vi "main.vi"() -> ()   [LabVIEW 2019]
uses:
  <vilib>/addons/Control Design/_Model Construction/Data Typedefs.llb/CD frequency specs.ctl
  <vilib>/addons/Control Design/_Frequency Response Analysis/Frequency Response.llb/Frequency Response subVI/cd_Bode (State Space).vi
  <vilib>/addons/Control Design/_Frequency Response Analysis/NI_CD_Frequency Response.lvlib
  <vilib>/addons/Control Design/_Model Construction/NI_LinSys_Data Typedefs.lvlib
panel:
  in  "As":dbl=5.0 caption="Амплитуда сигнала, As"
  out "АЧХ, вычисленный вручную":cluster{"Frequency":dbl[], dbl[]}(graph)
  out "Искомый массив частот":dbl[](array[numeric])=[1.0, 1.0473708979594496, 1.0969857978923836, 1.1489510001873091, 1.20337784077759, 1.2603829296797278, 1.3200884008314184, 1.3826221737646567, 1.4481182276745346, 1.5167168884709241, 1.5885651294280543, 1.6638168860761304, 1.7426333860096521, 1.8251834943190455, 1.9116440753857047, 2.0022003718155874, 2.0970464013232357, 2.1963853724165494, 2.3004301197729218, 2.409403560239529, 2.5235391704347703, 2.6430814869741095, 2.7682866303920703, 2.8994228538828817, 3.036771118035464, 3.180625692794125, 3.331294787934679, 3.489101213406779, 3.654383070957264, 3.8274944785163205, 4.008806328898474, 4.198707084443918, 4.397603609302729, 4.605922041145116, 4.824108704165382, 5.052631065335692, 5.291978735958455, 5.54266452066312, 5.805225516094915, 6.08022426164944, 6.368249944718606, 6.669919663030142, 6.98587974678527, 7.31680714342722, 7.663410868007483, 8.026433522257202, 8.406652885618355, 8.804883581643494, 9.22197882333436, 9.65883224115874, 10.11637979766211, 10.5956017927762, 11.097524964120764, 11.623224686798574, 12.173827277396665, 12.750512407130188, 13.354515629299048, 13.987131026472447, 14.649713983072926, 15.343684089300197, 16.070528182616467, 16.83180353330965, 17.629141180959564, 18.46424942895553, 19.33891750455241, 20.255019392306775, 21.21451784910641, 22.219468609395356, 23.272024789604217, 24.37444150122234, 25.529080682395318, 26.738416158399623, 28.005038941836467, 29.331662783900615, 30.721129988617754, 30.997000000000003, 32.176417502507555, 33.700643292719484, 35.29707302730671, 36.969127071950496, 38.72038781812579, 40.16172070631751, 40.32654463353467, 40.49204499907432, 40.55460735840854, 40.65822457904315, 40.82508616094098, 40.99263254370755, 41.160866537769486, 41.32979096508739, 41.499408659203226, 41.669722465287826, 41.840735240188614, 42.01244985247753, 42.18486918249916, 42.357996122419046, 42.47571552536925, 42.53183357627216, 42.706384460011684, 42.88165170155787, 43.05763824084719, 43.23434702988161, 43.41178103277815, 43.58994322581855, 43.76883659749926, 43.94846414858153, 44.12882889214174, 44.30993385362195, 44.48782831127613, 44.491782070880674, 44.67437659424378, 44.85772048655573, 45.04181682323088, 45.226668692305125, 45.41227919448768, 45.598651443213065, 45.78578856469338, 45.973693697970695, 46.162369994969744, 46.351820620550775, 46.54204875256262, 46.595256686647105, 46.73305758189605, 46.92485031253724, 47.11743016162157, 47.310800359487544, 47.504964149730995, 47.6999247892595, 47.895685548347, 48.09224971068864, 48.289620573455906, 48.48780144735186, 48.68679565666673, 48.80251583654462, 48.88660653933364, 49.087237446984595, 49.28869174500675, 49.4909728125988, 49.69408404282771, 49.8980288426856, 50.102810633146895, 50.30843284922574, 50.51489894003359, 50.72221236883706, 50.930376613116046, 51.114334834402, 51.13939516462204, 51.349271529436685, 51.56000922803062, 51.771611795322514, 51.984082780738355, 52.197425748271, 52.41164427653995, 52.62674195885138, 52.84272240325842, 53.05958923262166, 53.277346084669944, 53.495996612061354, 53.5356667741076, 53.71554448244452, 53.93599337852012, 54.15734699810265, 54.379609054182474, 54.60278327498806, 54.82687340404857, 55.051883200256626, 55.27781643793134, 55.50467690688171, 55.732468412470084, 55.96119477567605, 56.07169938205495, 56.1908598331605, 56.421467437330044, 56.65302145640156, 56.88552577446712, 57.11898429155914, 57.35340092371575, 57.58877960304659, 57.825124277798636, 58.062438912422536, 58.300727487639044, 58.539994000505814, 58.727866131895205, 58.780242464484466, 59.021476909507854, 59.263701382047735, 59.50691994518259, 59.751136678665794, 59.99635567899408, 60.24258105947626, 60.994, 61.509857885805424, 64.42363508721417, 67.4754405311074, 70.6718127392754, 74.01959996915694, 77.52597488629515, 81.19844993184068, 85.04489341802739, 89.07354638610502, 90.99100000000001, 93.2930402628475, 97.71241535346567, 102.34114021054606, 107.18913192051356, 112.2667773510822, 117.58495540521655, 120.988, 123.1550603292835, 128.98902612533183, 135.0993521198037, 141.4991297434587, 148.202070579887, 155.222535742706, 162.5755666443807, 170.27691722259138, 178.34308769319242, 186.7913599020798, 195.63983435170803, 204.90746898158642, 214.61411978584223, 224.78058335487444, 235.42864143224375, 246.58110758226243, 258.2618760682698, 270.4959730463159, 283.309610183935, 296.73024081888957, 310.7866187782041, 325.5088599835088, 340.9285069746843, 357.0785964900496, 373.99373024788326, 391.7101490809297, 410.2658105827232, 429.70047043208825, 450.0557675700542, 471.3753134116769, 493.7047852839051, 517.0920242896809, 541.5871378079527, 567.2426068492035, 594.1133984965093, 622.2570836730293, 651.7339604882491, 682.6071834272459, 714.9428986597652, 748.81038575901, 784.2822061337762, 821.4343584919513, 860.3464416684594, 901.1018251665116, 943.7878277775483, 988.4959046625692, 1035.3218432956735, 1084.3659686896222, 1135.7333583431182, 1189.5340673703329, 1245.8833642950221, 1304.9019780144174, 1366.716356462022, 1431.4589375234953, 1499.2684327860632, 1570.2901247293955, 1644.676177994683, 1722.5859653988068, 1804.1864093920938, 1889.6523396912323, 1979.166867853581, 2072.9217795953964, 2171.1179456945306, 2273.965752357956, 2381.685551976188, 2494.5081352303473, 2612.675225563361, 2736.439997074705, 2866.0676169482877, 3001.835813575628, 3144.0354715915405, 3292.9712550971935, 3448.962260405803, 3612.342699709479, 3783.462617131979, 3962.6886387015306, 4150.404757850531, 4347.013158125083, 4552.93507486701, 4768.611697714535, 4994.505115855208, 5231.099308056334, 5478.901179594018, 5738.441648302474, 6010.276782070467, 6294.988990221976, 6593.18827133364, 6905.513520162426, 7232.6338964836405, 7575.250258772024, 7934.096665797607, 8309.941949353515, 8703.591361485289, 9115.888299750955, 9547.716114208199, 9850.015, 9880.012, 9910.009, 9940.006, 9970.003, 10000.0]
  out "АЧХ":cluster{"W":dbl[], "Magnitude":dbl[]}[](graph)
  in  "t, [s]":dbl=1.0 caption="Время t, [s]"
  in  "An":dbl caption="Амплитуда шума, An"
  in  "dt [s]":dbl=0.001 caption="Шаг дискретизации dt [s]"
  in  "f, [Hz]":dbl=1.0 caption="Частота сигнала f, [Hz]"
  in  "f_cut":dbl=10.0 caption="Частота среза f_cut [Hz]"
  in  "dbs":dbl=120.0 caption="Пульсации в полосе\nпропускания dbs, [db]"
  in  "dbp":dbl=0.05 caption="Пульсации в полосе\nподавления dbp [db]"
  in  "n":i32=2 caption="Порядок фильтра n"
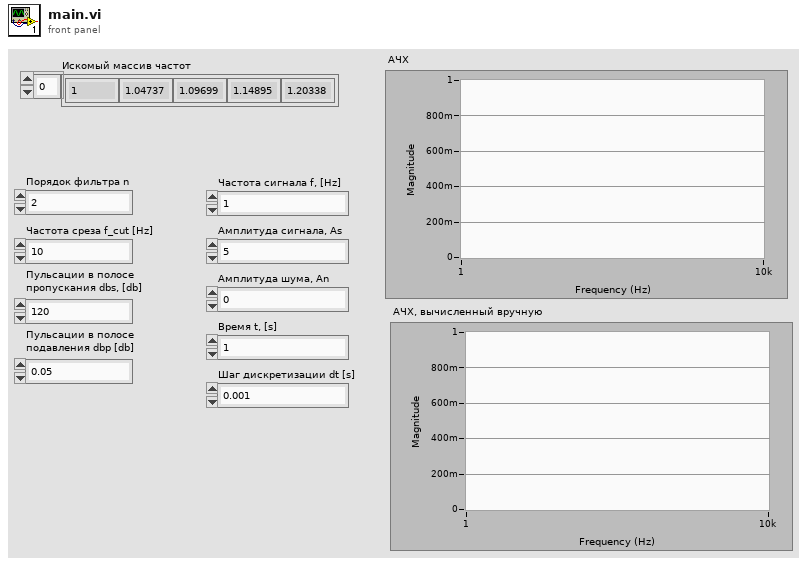
[diagram p1: front panel]
types:
  T1 = typedef "NI_LinSys_Data Typedefs.lvlib/CD frequency specs.ctl" = cluster{"Initial frequency":dbl, "Final frequency":dbl, "Minimum number of points":i32, "Frequency Unit":enum16{"Hz", "rad/s"}}
  T2 = typedef "NI_LinSys_Model Typedefs.lvlib/CD State Space Model (MIMO).ctl" = cluster{"properties":T3, "A":dbl[][], "B":dbl[][], "C":dbl[][], "D":dbl[][], "StateNames":string[], "Transport Delay":dbl[][]}
  T3 = typedef "NI_LinSys_Model Typedefs.lvlib/CD General Elements.ctl" = cluster{"Model name":string, "Input names":string[], "Output names":string[], "Input Delays":dbl[], "Output Delays":dbl[], "Sampling Time":dbl, "Notes":string}
  T4 = typedef "NI_LinSys_Data Typedefs.lvlib/CD Bode Data.ctl" = cluster{"Frequency":dbl[], "Magnitude":dbl[][][], "Phase":dbl[][][], "plot type":T5}
  T5 = typedef "NI_LinSys_Data Typedefs.lvlib/CD Plot Types Enum.ctl" = enum16{"bode-magnitude", "bode-phase", "nichols", "nyquist", "singular values", "step", "impulse", "initial", "simulation", "nyquist with separation"}
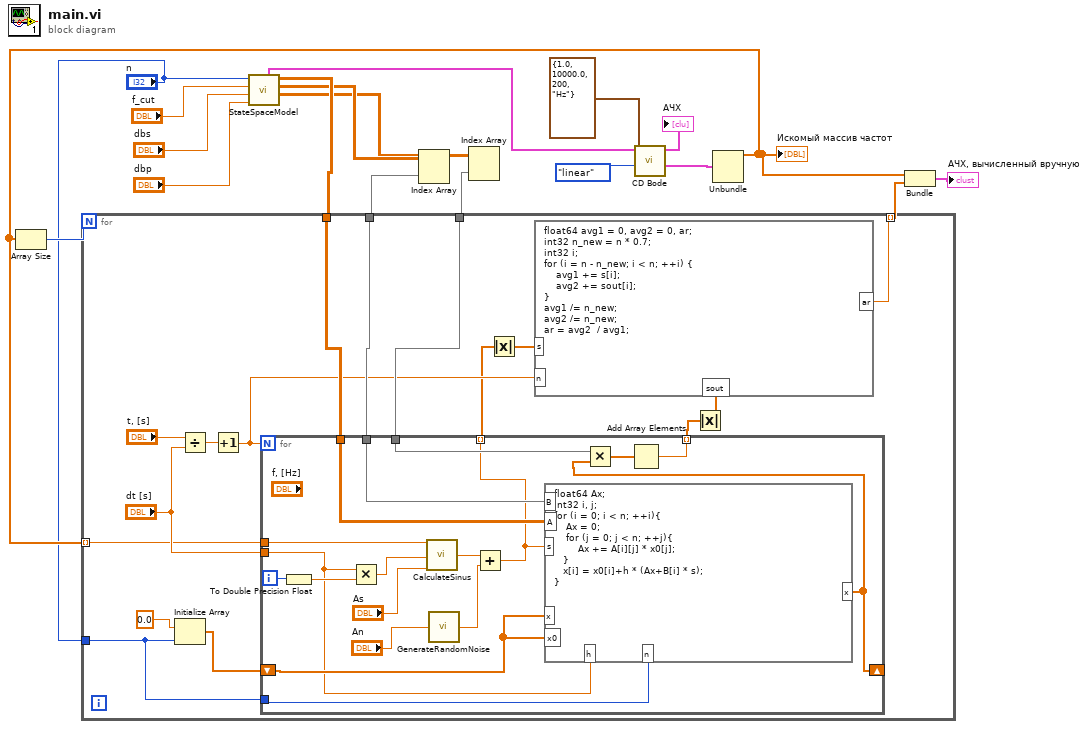
[diagram p0: block diagram]
diagram:
  n1 = call "StateSpaceModel.vi"("dbp"="dbp", "dbs"="dbs", "f_cut"="f_cut", "n"="n") -> ("C"=w2:dbl[][], "B"=w3:dbl[][], "A"=w4:dbl[][], "State-Space Model"=w1:T2)  [unwired: 1 in, 1 out]
  n2 = Index Array(array=w3) -> (element=w18:dbl[])  [unwired: 2 in]
  n3 = Index Array(array=w2) -> (element=w17:dbl[])  [unwired: 2 in]
  n4 = call-poly <vilib>:"CD Bode.vi"("Magnitude Scale"=enum16{"linear", "dB"}."linear", "Frequency Range"=T1 {"Initial frequency"=1.0, "Final frequency"=10000.0, "Minimum number of points"=200, "Frequency Unit"=enum."Hz"}, "State-Space Model"=w1) -> ("Bode Data"=w14:T4, "Bode Magnitude"=→"АЧХ":cluster{"W":dbl[], "Magnitude":dbl[]}[])  [unwired: 4 in, 3 out]
  n5 = Unbundle(w14) -> ("Frequency"=w11:dbl[])  [unwired: 3 out]
  "Искомый массив частот" <- w11
  n6 = Array Size(array=w11) -> (size(s)=w12:i32)
  n7 = for {
    N: w12 -> [_]
    tunnel: w4 -> [w34]
    tunnel: w18 -> [w33]
    tunnel: w17 -> [w27]
    tunnel: "n" -> [w26]
    tunnel: [w21] -> w10 mode=indexing
    tunnel: w11 -> [w19] mode=indexing
    n8 = Initialize Array(0.0, w26) -> (w28:dbl[])
    n9 = Divide(x="t, [s]", y="dt [s]") -> (x/y=w30:dbl)
    n10 = Increment(x=w30) -> (x+1=w25:dbl)
    n11 = for {
      N: w25 -> [_]
      tunnel: w34 -> [w51]
      tunnel: w33 -> [w50]
      tunnel: "dt [s]" -> [w40]
      shift-right: [w35] -> _
      shift-left: w28 -> [w45]
      tunnel: w27 -> [w49]
      tunnel: [w48] -> w20 mode=indexing
      tunnel: [w46] -> w23 mode=indexing
      tunnel: w26 -> [w44]
      tunnel: w19 -> [w39]
      i -> [w52]
      n12 = To Double Precision Float(number=w52) -> (double precision float=w41:dbl)
      n13 = Multiply(x=w40, y=w41) -> (x*y=w38:dbl)
      n14 = call "CalculateSinus.vi"("As"="As", "t, [s]"=w38, "f, [Hz]"=w39) -> ("Значение синуса"=w36:dbl)
      n15 = call "GenerateRandomNoise.vi"("An"="An") -> ("Шум"=w42:dbl)
      n16 = Add(x=w36, y=w42) -> (x+y=w48:dbl)
      n17 = formula code="float64 Ax;\nint32 i, j;\nfor (i = 0; i < n; ++i){\n    Ax = 0;\n    for (j = 0; j < n; ++j){\n        Ax += A[i][j] * x0[j];\n   }\n   x[i] = x0[i]+h * (Ax+B[i] * s);\n}"("B"=w50, "A"=w51, "s"=w48, "x"=w45, "x0"=w45, "n"=w44, "h"=w40) -> ("x"=w35:dbl[])
      n18 = Multiply(x=w49, y=w35) -> (x*y=w47:dbl[])
      n19 = Add Array Elements(numeric array=w47) -> (sum=w46:dbl)
    }
    n20 = Absolute Value(x=w20) -> (abs(x)=w22:dbl[])
    n21 = Absolute Value(x=w23) -> (abs(x)=w24:dbl[])
    n22 = formula code="float64 avg1 = 0, avg2 = 0, ar;\nint32 n_new = n * 0.7;\nint32 i;\nfor (i = n - n_new; i < n; ++i) {\n    avg1 += s[i];\n    avg2 += sout[i];\n}\navg1 /= n_new;\navg2 /= n_new;\nar = avg2  / avg1;"("n"=w25, "s"=w22, "sout"=w24) -> ("ar"=w21:dbl)
  }
  n23 = Bundle("Frequency"=w11, w10) -> (→"АЧХ, вычисленный вручную":cluster{"Frequency":dbl[], dbl[]})  [unwired: 1 in]
